vi "LEDSA --UP--.vi"(2 "Error In":errorcluster, 3 "FPGA VI Reference In":refnum<k20>) -> (0 "Error Out":errorcluster, 1 "FPGA VI Reference Out":refnum<k20>)   [LabVIEW 2015]
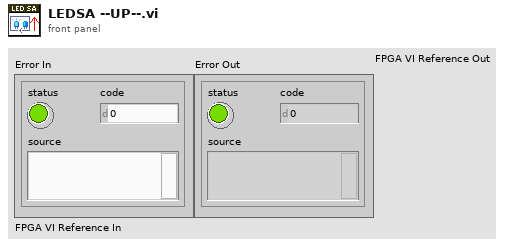
[diagram p1: front panel]
types:
  T1 = cluster{"LED 3":enum16{"Brightness", "Bool"}, "BOOL":bool, "Brightness":u32}
  T2 = cluster{"LED 1":enum16{"Brightness", "Bool"}, "BOOL":bool, "Brightness":u32}
  T3 = cluster{"LED 2":enum16{"Brightness", "Bool"}, "BOOL":bool, "Brightness":u32}
  T4 = cluster{"LED 0":enum16{"Brightness", "Bool"}, "BOOL":bool, "Brightness":u32}
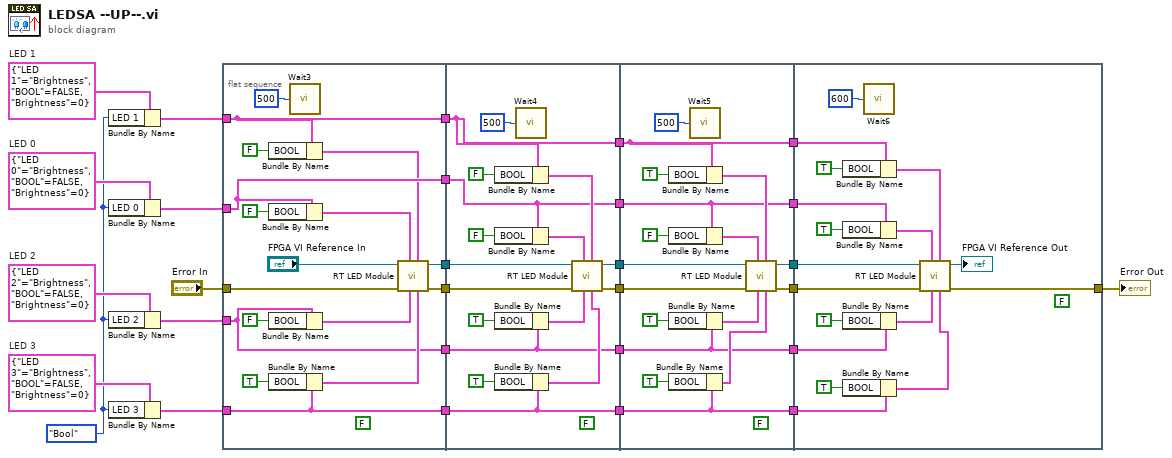
[diagram p0: block diagram]
diagram:
  w21 = T1 {"LED 3"=enum."Brightness", "BOOL"=FALSE, "Brightness"=0}  # LED 3
  w24 = T2 {"LED 1"=enum."Brightness", "BOOL"=FALSE, "Brightness"=0}  # LED 1
  w22 = T3 {"LED 2"=enum."Brightness", "BOOL"=FALSE, "Brightness"=0}  # LED 2
  w23 = T4 {"LED 0"=enum."Brightness", "BOOL"=FALSE, "Brightness"=0}  # LED 0
  w20 = enum16{"Brightness", "Bool"}."Bool" ("LED")
  n1 = Bundle By Name(cluster=w24, "LED 1"=w20) -> (w6:T2)
  n2 = Bundle By Name(cluster=w23, "LED 0"=w20) -> (w7:T4)
  n3 = Bundle By Name(cluster=w22, "LED 2"=w20) -> (w5:T3)
  n4 = Bundle By Name(cluster=w21, "LED 3"=w20) -> (w4:T1)
  n5 = flat-sequence {
    tunnel: [w46] -> w29
    tunnel: "Error In" -> [w44]
    tunnel: [w40] -> w19
    tunnel: [w38] -> w16
    tunnel: [w37] -> w13
    tunnel: [w36] -> w10
    tunnel: w7 -> [w40]
    tunnel: w6 -> [w38]
    tunnel: w5 -> [w37]
    tunnel: w4 -> [w36]
    tunnel: [w31] -> w3
    tunnel: w29 -> [w62]
    tunnel: [w63] -> w28
    tunnel: w19 -> [w56]
    tunnel: [w56] -> w18
    tunnel: w16 -> [w55]
    tunnel: [w55] -> w15
    tunnel: w13 -> [w54]
    tunnel: [w54] -> w12
    tunnel: w10 -> [w53]
    tunnel: [w53] -> w9
    tunnel: w3 -> [w48]
    tunnel: [w47] -> w2
    tunnel: w28 -> [w79]
    tunnel: [w80] -> w27
    tunnel: w18 -> [w73]
    tunnel: [w73] -> w17
    tunnel: w15 -> [w72]
    tunnel: [w72] -> w14
    tunnel: w12 -> [w71]
    tunnel: [w71] -> w11
    tunnel: w9 -> [w70]
    tunnel: [w70] -> w8
    tunnel: w2 -> [w65]
    tunnel: [w64] -> w1
    tunnel: [w97] -> w25
    tunnel: w27 -> [w96]
    tunnel: w17 -> [w90]
    tunnel: w14 -> [w89]
    tunnel: w11 -> [w88]
    tunnel: w8 -> [w87]
    tunnel: w1 -> [w82]
    frame #0 {
      (unwired) FALSE ("Stop Button")
      n6 = Bundle By Name(cluster=w38, "BOOL"=FALSE) -> (w39:T2)
      n7 = Bundle By Name(cluster=w40, "BOOL"=FALSE) -> (w43:T4)
      n8 = Bundle By Name(cluster=w37, "BOOL"=FALSE) -> (w42:T3)
      n9 = Bundle By Name(cluster=w36, "BOOL"=TRUE) -> (w41:T1)
      n10 = call "Wait3"("Count(mSec)"=u32 500) -> ()  [unwired: 1 out]
      n11 = call "RT LED Module.vi"("LED 3"=w41, "LED 1"=w39, "LED 2"=w42, "LED 0"=w43, "error in"=w44, "FPGA VI Reference In"="FPGA VI Reference In") -> ("error out"=w46:errorcluster, "FPGA VI Reference Out"=w31:refnum<k20>)  [unwired: 4 in]
    }
    frame #1 {
      (unwired) FALSE ("Stop Button")
      n12 = Bundle By Name(cluster=w55, "BOOL"=FALSE) -> (w60:T2)
      n13 = Bundle By Name(cluster=w56, "BOOL"=FALSE) -> (w59:T4)
      n14 = Bundle By Name(cluster=w54, "BOOL"=TRUE) -> (w57:T3)
      n15 = Bundle By Name(cluster=w53, "BOOL"=TRUE) -> (w58:T1)
      n16 = call "Wait4"("Count(mSec)"=u32 500) -> ()  [unwired: 1 out]
      n17 = call "RT LED Module.vi"("LED 3"=w58, "LED 1"=w60, "LED 2"=w57, "LED 0"=w59, "error in"=w62, "FPGA VI Reference In"=w48) -> ("error out"=w63:errorcluster, "FPGA VI Reference Out"=w47:refnum<k20>)  [unwired: 4 in]
    }
    frame #2 {
      (unwired) FALSE ("Stop Button")
      n18 = Bundle By Name(cluster=w72, "BOOL"=TRUE) -> (w75:T2)
      n19 = Bundle By Name(cluster=w73, "BOOL"=FALSE) -> (w74:T4)
      n20 = Bundle By Name(cluster=w71, "BOOL"=TRUE) -> (w76:T3)
      n21 = Bundle By Name(cluster=w70, "BOOL"=TRUE) -> (w77:T1)
      n22 = call "Wait5"("Count(mSec)"=u32 500) -> ()  [unwired: 1 out]
      n23 = call "RT LED Module.vi"("LED 3"=w77, "LED 1"=w75, "LED 2"=w76, "LED 0"=w74, "error in"=w79, "FPGA VI Reference In"=w65) -> ("error out"=w80:errorcluster, "FPGA VI Reference Out"=w64:refnum<k20>)  [unwired: 4 in]
    }
    frame #3 {
      (unwired) FALSE ("Stop Button")
      n24 = Bundle By Name(cluster=w89, "BOOL"=TRUE) -> (w93:T2)
      n25 = Bundle By Name(cluster=w90, "BOOL"=TRUE) -> (w94:T4)
      n26 = Bundle By Name(cluster=w88, "BOOL"=TRUE) -> (w92:T3)
      n27 = Bundle By Name(cluster=w87, "BOOL"=TRUE) -> (w91:T1)
      n28 = call "Wait6"("Count(mSec)"=u32 600) -> ()  [unwired: 1 out]
      n29 = call "RT LED Module.vi"("LED 3"=w91, "LED 1"=w93, "LED 2"=w92, "LED 0"=w94, "error in"=w96, "FPGA VI Reference In"=w82) -> ("error out"=w97:errorcluster, "FPGA VI Reference Out"=→"FPGA VI Reference Out":refnum<k20>)  [unwired: 4 in]
    }
  }
  "Error Out" <- w25
